vi "Commit Buffer.vi"(7 "Action":T1, 8 "error in (no error)":errorcluster, 9 "Transation String":string, 11 "device name in":string) -> (0 "error out":errorcluster, 1 "Transactions":string[](array[string]))   [LabVIEW 2015, in "SLSC Switch.lvlib" / "RelayInterface.lvclass"]
uses:
  RelayInterface.lvclass
  Commit Buffer Action.ctl
  Session Transaction Buffer.ctl
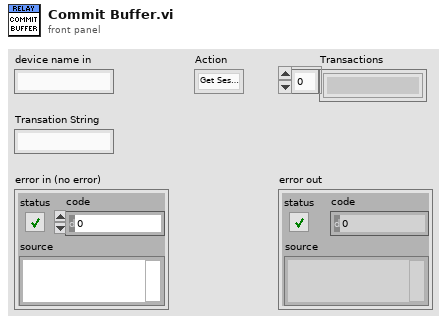
[diagram p1: front panel]
types:
  T1 = typedef "SLSC Switch.lvlib/RelayInterface.lvclass/Commit Buffer Action.ctl" = enum16{"Get Session Buffer", "Add Transaction", "Clear Session Buffer", "Clear All"}
  T2 = typedef "SLSC Switch.lvlib/RelayInterface.lvclass/Session Transaction Buffer.ctl" = cluster{"buffer id":string, "Transactions":string[]}
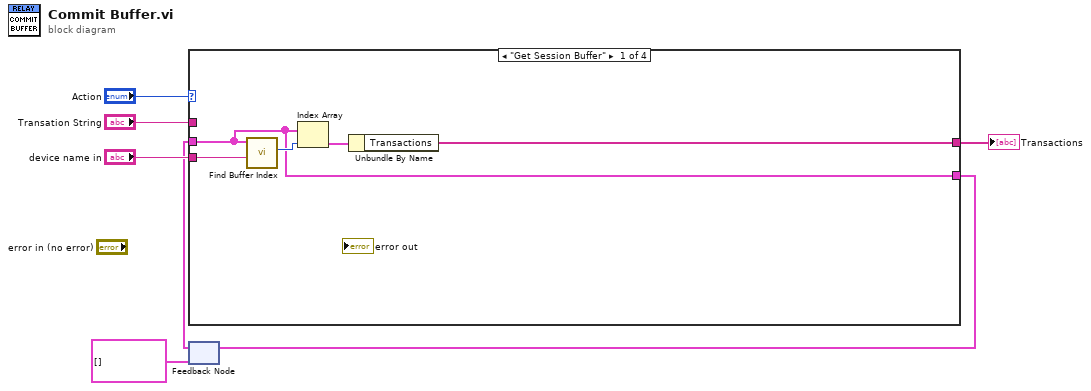
[diagram p0: block diagram]
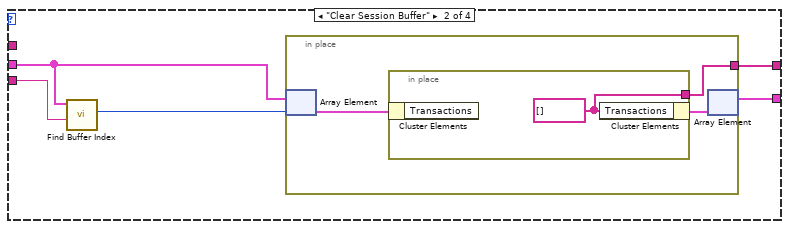
[diagram p2: hidden frame]
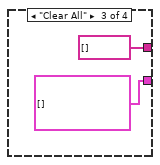
[diagram p3: hidden frame]
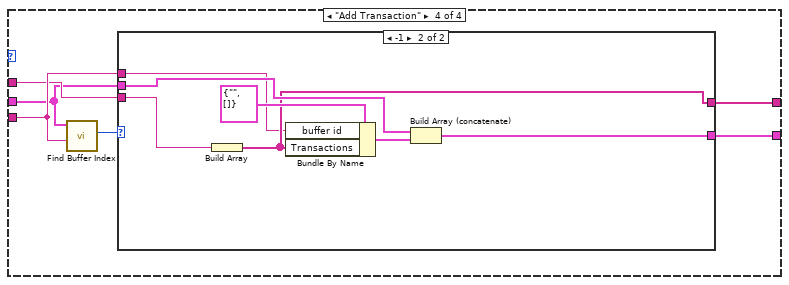
[diagram p4: hidden frame]
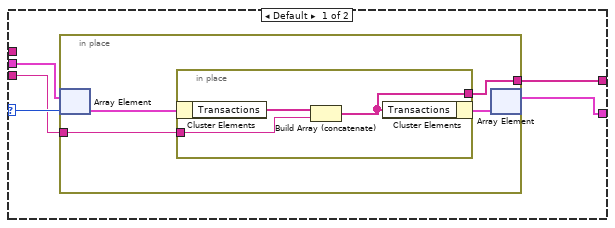
[diagram p5: hidden frame]
diagram:
  n1 = feedback #1(T2[] [] ("Session Transaction Buffers")) -> (w3:T2[])
  n2 = case shown="\"Get Session Buffer\"" "Action" {
    tunnel: "Transation String" -> [_ _ _ w27]
    tunnel: "device name in" -> [w8 w17 _ w28]
    tunnel: w3 -> [w9 w15 _ w26]
    tunnel: [w10 w13 string[] [] ("Transactions") w24] -> w2
    tunnel: [w9 w14 T2[] [] ("Session Transaction Buffers") w25] -> w1
    frame "Get Session Buffer" {
      n3 = call "Find Buffer Index.vi"("buffer id"=w8, "Session Transaction Buffers"=w9) -> ("index"=w12:i32)  [unwired: 9 in]
      n4 = Index Array(array=w9, index=w12) -> (element=w11:T2)
      n5 = Unbundle By Name(w11) -> ("Transactions"=w10:string[])
    }
    frame "Clear Session Buffer" {
      n6 = call "Find Buffer Index.vi"("buffer id"=w17, "Session Transaction Buffers"=w15) -> ("index"=w16:i32)  [unwired: 9 in]
      n7 = in-place {
        in-place-border: [w18] -> w13
        n8 = in-place-array #2(w15, w16) -> (w20:T2)
        n9 = in-place {
          in-place-border: [w21] -> w18
          w21 = string[] [] ("Transactions")
          n10 = in-place-cluster #3(w20) -> ()  [unwired: 1 out]
          n11 = in-place-cluster #3("Transactions"=w21) -> (w19:T2)
        }
        n12 = in-place-array #2(w19) -> (w14:T2[])  [unwired: 1 out]
      }
    }
    frame "Clear All" {
    }
    frame "Add Transaction" {
      n13 = call "Find Buffer Index.vi"("buffer id"=w28, "Session Transaction Buffers"=w26) -> ("index"=w29:i32)  [unwired: 9 in]
      n14 = case shown="-1" w29 {
        selector: w29 -> [w33 _]
        tunnel: w28 -> [_ w42]
        tunnel: w27 -> [w31 w47]
        tunnel: w26 -> [w34 w45]
        tunnel: [w32 w44] -> w25
        tunnel: [w30 w43] -> w24
        frame Default {
          n15 = in-place {
            in-place-border: w31 -> [w37]
            in-place-border: [w35] -> w30
            n16 = in-place-array #4(w34, w33) -> (w38:T2)
            n17 = in-place {
              in-place-border: w37 -> [w41]
              in-place-border: [w39] -> w35
              n18 = in-place-cluster #5(w38) -> ("Transactions"=w40:string[])
              n19 = Build Array (concatenate)(w40, w41) -> (w39:string[])
              n20 = in-place-cluster #5("Transactions"=w39) -> (w36:T2)
            }
            n21 = in-place-array #4(w36) -> (w32:T2[])  [unwired: 1 out]
          }
        }
        frame -1 {
          n22 = Build Array(w47) -> (w43:string[])
          n23 = Bundle By Name(cluster=T2 {"buffer id"="", "Transactions"=[]} ("Session Transaction Buffer"), "buffer id"=w42, "Transactions"=w43) -> (w46:T2)
          n24 = Build Array (concatenate)(w45, w46) -> (w44:T2[])
        }
      }
    }
  }
  "Transactions" <- w2
  n25 = feedback-in #1(w1) -> ()
